vi "PicoScope2000aGetTimebase2.vi"(4 "Number of Samples":u32, 6 "Memory Segment":u32, 7 "Acquisition Settings":T1={"preTriggerSamples"=0, "postTriggerSamples"=5000000, "timebase"=5} {"postTriggerSamples" format="%_6p"; "preTriggerSamples" format="%_6p"}, 8 "error in (no error)":errorcluster, 11 "handle in":i16) -> (0 "error out":errorcluster, 3 "handle out":i16, 5 "Properties Panel":T2 {"Max Total Capture Time Available (sec)" format="%.3p"; "Sample Frequency" format="%.3p"; "Sample Internal" format="%.3p"; "Max Samples Available" format="%.3p"; "Total Capture Time (sec)" format="%.3p"})   [LabVIEW 2010]
uses:
  ps2000a.dll
  shared/Acquisition Settings.ctl
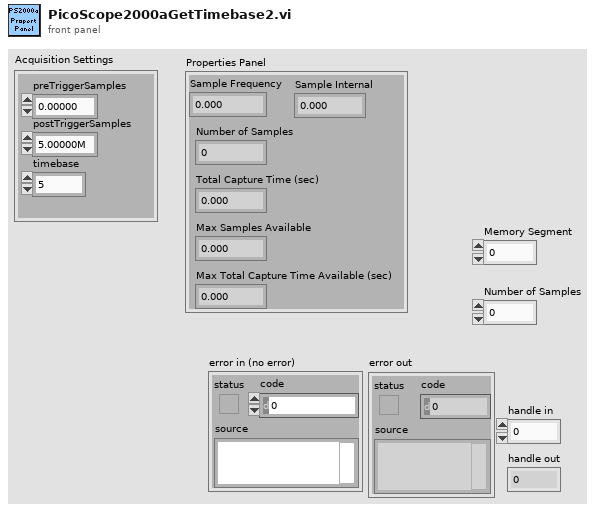
[diagram p1: front panel]
types:
  T1 = typedef "Acquisition Settings.ctl" = cluster{"preTriggerSamples":u64, "postTriggerSamples":u64, "timebase":u32}
  T2 = cluster{"Sample Frequency":sgl, "Sample Internal":sgl, "Max Samples Available":i32, "Number of Samples":u32, "Total Capture Time (sec) ":sgl, "Max Total Capture Time Available (sec)":sgl}
  T3 = cluster{sgl, sgl, "maxSamples":i32, "Number of Samples":u32, sgl, sgl}
  T4 = cluster{"status":bool, "code":u32, "source":string}
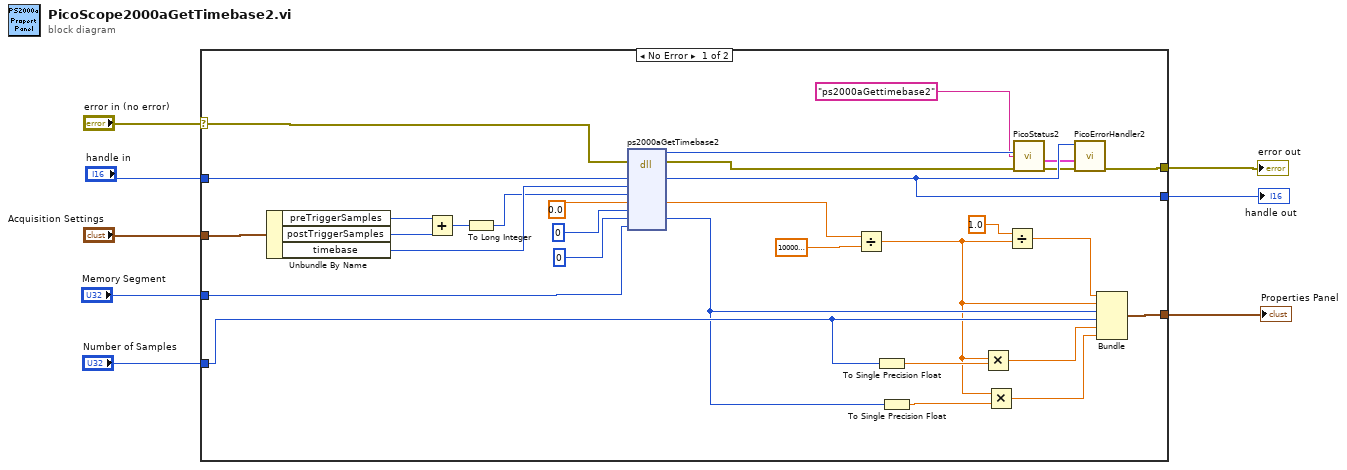
[diagram p0: block diagram]
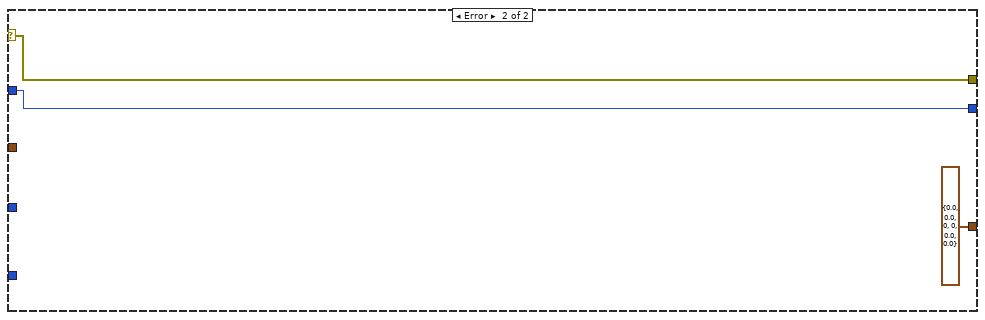
[diagram p2: hidden frame]
diagram:
  n1 = case shown="No Error" "error in (no error)" {
    selector: "error in (no error)" -> [w12 w40]
    tunnel: [w31 w42] -> w3
    tunnel: "Memory Segment" -> [w13 _]
    tunnel: "Number of Samples" -> [w26 _]
    tunnel: "handle in" -> [w30 w42]
    tunnel: "Acquisition Settings" -> [w29 _]
    tunnel: [w22 T3 {0.0, 0.0, "maxSamples"=0, "Number of Samples"=0, 0.0, 0.0}] -> w4
    tunnel: [w10 w40] -> w1
    frame No Error {
      n2 = Unbundle By Name(w29) -> ("preTriggerSamples"=w34:u64, "postTriggerSamples"=w35:u64, "timebase"=w36:u32)
      n3 = Add(x=w34, y=w35) -> (x+y=w15:u64)
      n4 = To Long Integer(number=w15) -> (32bit integer=w14:i32)
      n5 = dll-call lib="ps2000a.dll" fn="ps2000aGetTimebase2"(error in=w12, "handle"=w30, "timebase"=w36, "noSamples"=w14, "timeIntervalNanoseconds"=sgl 0.0, "oversample"=i16 0, "maxSamples"=0, "segmentIndex"=w13) -> (error out=w37:errorcluster, "PICO_STATUS"=w32:u32, "handle"=w31:i16, "timeIntervalNanoseconds"=w38:sgl, "maxSamples"=w24:i32)  [unwired: 6 in, 1 out]
      n6 = Divide(x=w38, y=sgl 1000000000.0) -> (x/y=w17:sgl)
      n7 = To Single Precision Float(number=w26) -> (single precision float=w28:sgl)
      n8 = To Single Precision Float(number=w24) -> (single precision float=w25:sgl)
      n9 = Multiply(x=w17, y=w28) -> (x*y=w27:sgl)
      n10 = Multiply(x=w17, y=w25) -> (x*y=w23:sgl)
      n11 = Divide(x=sgl 1.0, y=w17) -> (x/y=w18:sgl)
      n12 = call "PicoStatus2.vi"("PICO source"="ps2000aGettimebase2" ("source"), "Error in"=w37, "PICO STATUS"=w32) -> ("error out"=w11:errorcluster, "PICO_STATUS out"=w9:T4)  [unwired: 5 in]
      n13 = call "PicoErrorHandler2.vi"("error in (no error)"=w11, "PICO_STATUS in"=w9, "handle In"=w31) -> ("error out"=w10:errorcluster)  [unwired: 8 in]
      n14 = Bundle(w18, w17, "maxSamples"=w24, "Number of Samples"=w26, w27, w23) -> (w22:T3)  [unwired: 1 in]
    }
    frame Error {
    }
  }
  "error out" <- w1
  "handle out" <- w3
  "Properties Panel" <- w4
